vi "PDF Protokoll O2 Leaktest.vi"(8 "error in (no error)":errorcluster caption="Fehler (Eingang, kein Fehler)") -> (0 "error out":errorcluster caption="Fehler (Ausgang)")   [LabVIEW 2020, in "O2 Dichtheitstest.lvlib"]
uses:
  O2 Dichtheitstest.lvlib
  Seiten/System Einstellungen V2/Aktioen FGV System Konstanten.ctl
  Aktion FGV O2 Leak.ctl
  <vilib>/Utility/miscctls.llb/LVPrintingMarginsTypeDef.ctl
  Allgemein/allgemeine Sub-VIs.lvlib
  Seiten/System Einstellungen V2/System Einstellungen V2.lvlib
panel:
  out "Grenzwert Messgasdruck:":string
  out "Messgasdruck:":string
  out "Grenzwert O2:":string
  out "Bestanden":bool caption="Boolesch"
  out "Nullgas Messwert:":string
  out "Datenerfassungszeit:":string
  out "Nullgas Aufschaltzeit:":string
  out "Analysator:":string
  out "Aufschaltpunkt:":string
  out "Endzeit:":string
  out "Startzeit:":string
  out "Ser.Nr.:":string caption="Serien Nummer:"
  out "Messgerät:":string
  # "O2 Leaktest"
  # "s"
  # "s"
  # "kPa"
  # "%"
  # "IAG-Industrie Automatisierungsgeschellschaft m.b.H.    l  Industriestraße 2    l    2722Weikersdorf     )+43262221734 7+43262221734655"
  # "kPa"
  # "%"
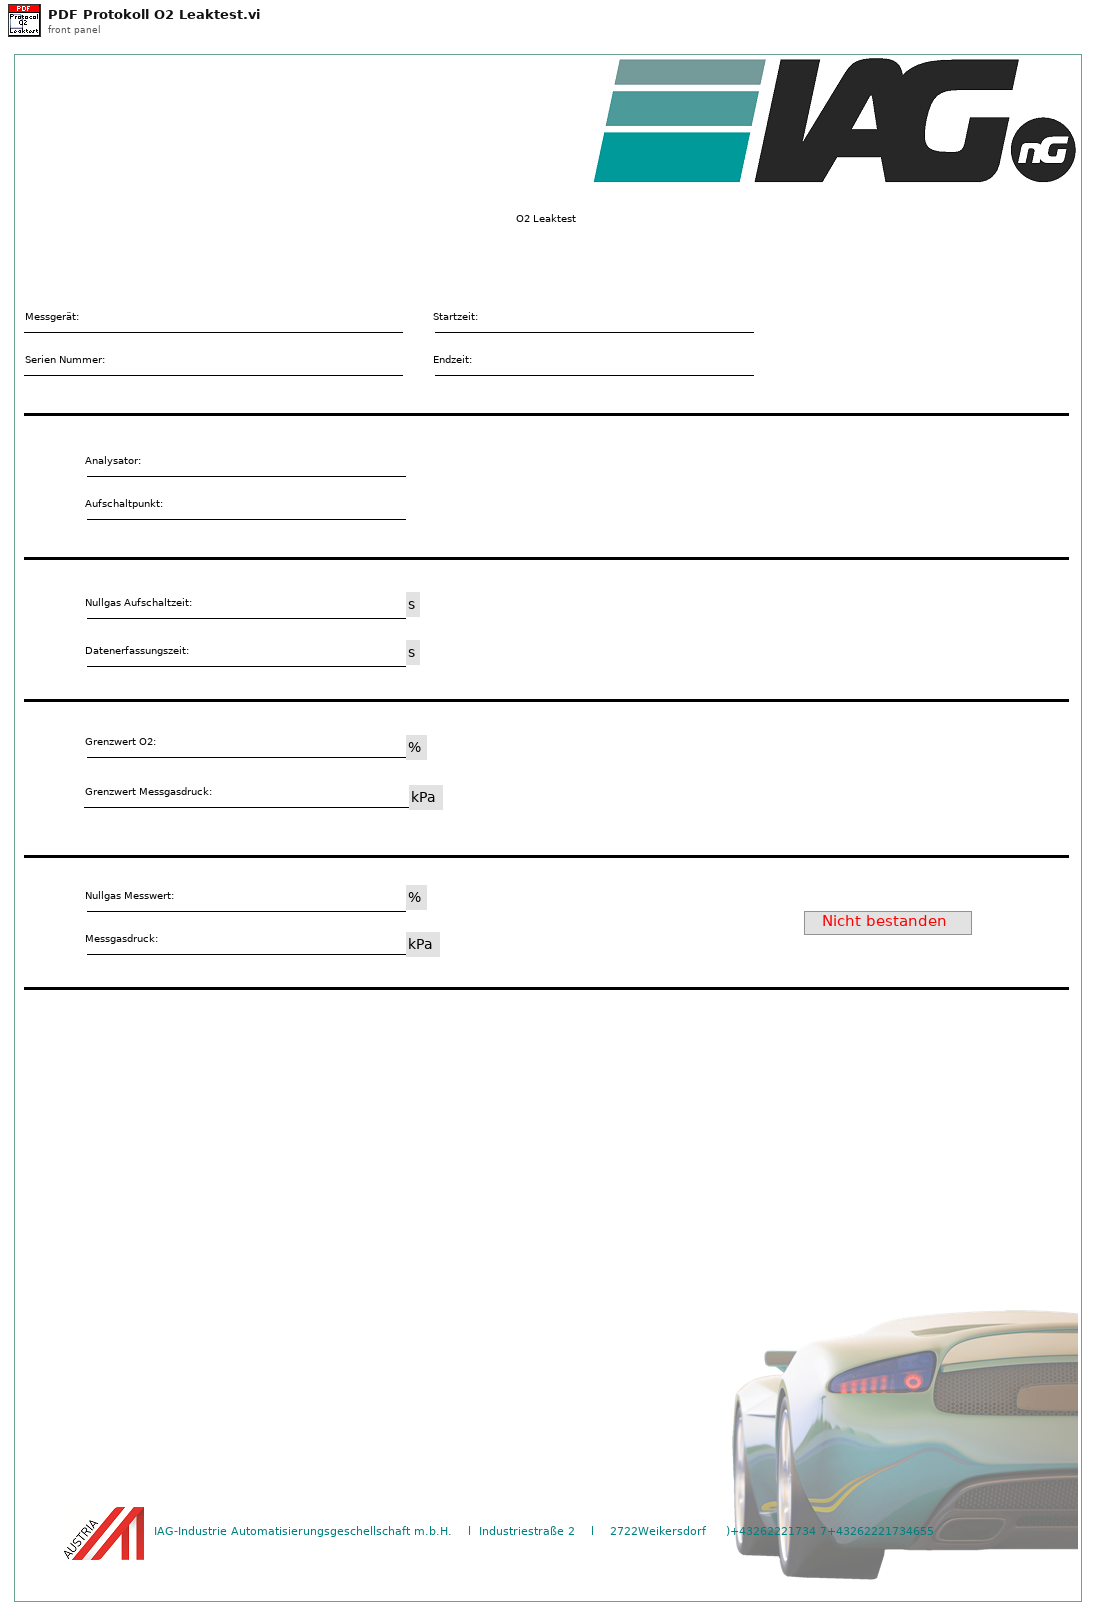
[diagram p1: front panel]
types:
  T1 = typedef "O2 Dichtheitstest.lvlib/Aktion FGV O2 Leak.ctl" = enum16{"lesen", "O2 settings", "Pfad", "Protokoll", "laden", "speichern"}
  T2 = typedef "System Einstellungen V2.lvlib/Aktioen FGV System Konstanten.ctl" = enum16{"lesen", "laden", "speichern", "Sprache"}
  T3 = enum32{"Portrait", "Landscape", "Rotated Portrait", "Rotated Landscape"}
  T4 = typedef "LVPrintingMarginsTypeDef.ctl" = cluster{"Top":sgl, "Left":sgl, "Bottom":sgl, "Right":sgl, "Measurement System":enum8{"Inches", "cm"}}
  T5 = typedef "O2 Dichtheitstest.lvlib/O2 Settings.ctl" = cluster{"Kalibriergas":T6, "Aufschaltpunkt":T6, "Nullgas Aufschaltzeit:":sgl, "Datenerfassungszeit:":sgl, "Grenzwert: O2":sgl, "Grenzwert: Messgasdruck":sgl, "Grenzwert: Messgasdruck 2":sgl}
  T6 = typedef "Auswahlfeld.ctl" = u16
  T7 = typedef "O2 Dichtheitstest.lvlib/Protokoll LeakTest.ctl" = cluster{"O2":sgl, "Messgasdruck":sgl, "Startzeit":timestamp, "Endzeit":timestamp, "Bestanden?":bool}
  T8 = cluster{"Modell":string, "ProjektNummer":string, "Software Version":string, "Seriennummer":string}
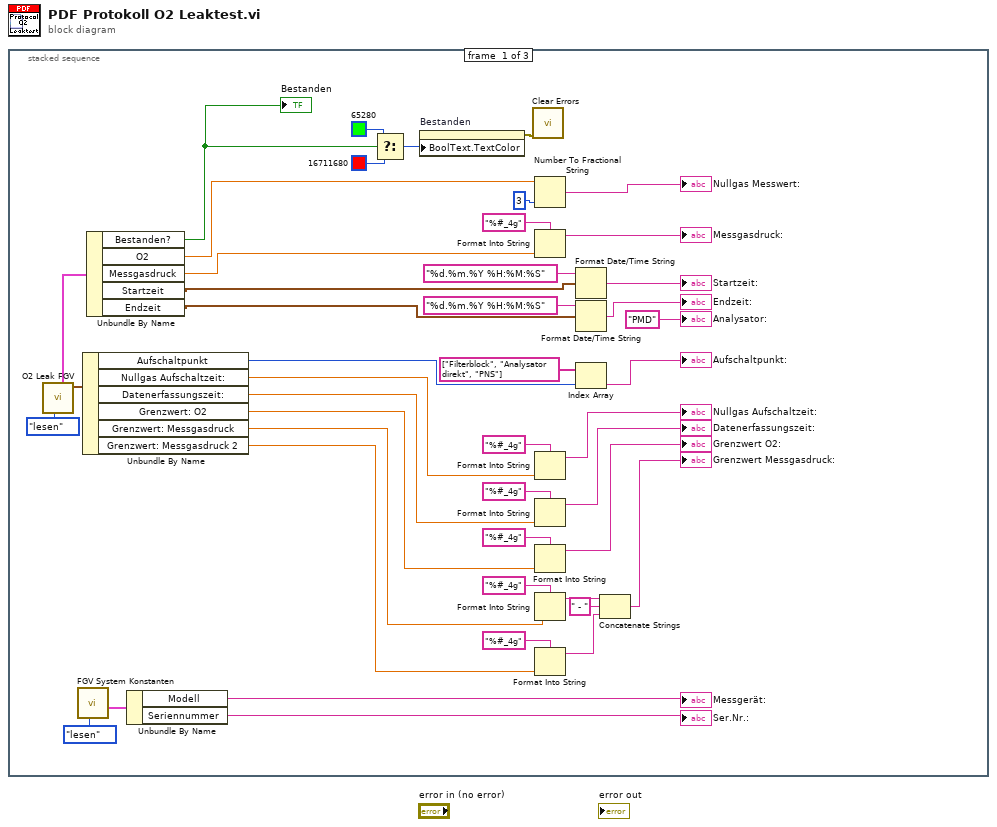
[diagram p0: block diagram]
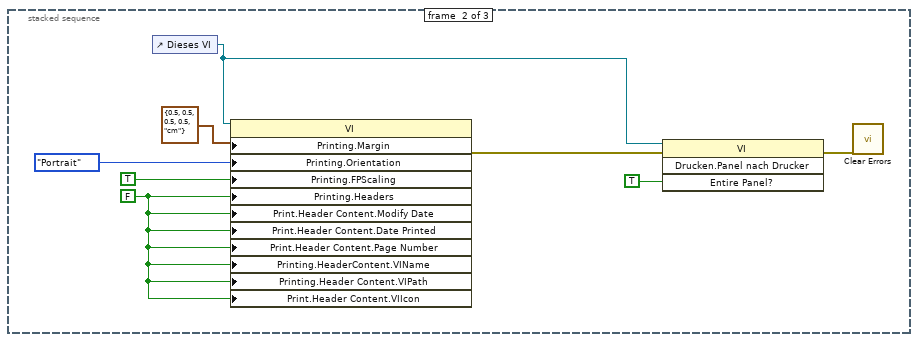
[diagram p2: hidden frame]
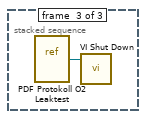
[diagram p3: hidden frame]
diagram:
  n1 = stacked-sequence {
    frame #0 {
      n2 = call "O2 Leak FGV.vi"("Aktion"=Aktion_FGV_O2_Leak."lesen") -> ("O2 Settings"=w17:T5, "Protokoll"=w18:T7)  [unwired: 6 in, 3 out]
      n3 = call "FGV System Konstanten.vi"("Aktionen"=Aktioen_FGV_System_Konstanten."lesen") -> ("Cluster out"=w44:T8)  [unwired: 6 in, 4 out]
      n4 = Unbundle By Name(w17) -> ("Aufschaltpunkt"=w14:T6, "Nullgas Aufschaltzeit:"=w12:sgl, "Datenerfassungszeit:"=w11:sgl, "Grenzwert: O2"=w10:sgl, "Grenzwert: Messgasdruck"=w9:sgl, "Grenzwert: Messgasdruck 2"=w7:sgl)
      n5 = Unbundle By Name(w18) -> ("Bestanden?"=w8:bool, "O2"=w1:sgl, "Messgasdruck"=w13:sgl, "Startzeit"=w16:timestamp, "Endzeit"=w15:timestamp)
      "Bestanden" <- w8
      n6 = Unbundle By Name(w44) -> ("Modell"=→"Messgerät:":string, "Seriennummer"=→"Ser.Nr.:":string)
      n7 = Select(t=u32 65280, s=w8, f=u32 16711680) -> (s? t:f=w21:u32)
      n8 = property on="Bestanden" class="Bool. (strikt)"("BoolText.TextColor"=w21) -> (error out=w20:errorcluster)  [unwired: 2 in, 1 out]
      n9 = call <vilib>:"Clear Errors.vi"("error in (no error)"=w20) -> ()  [unwired: 5 in, 2 out]
      n10 = Number To Fractional String(number=w1, precision (6)=i16 3 ("Breite (-)")) -> (F-format string=→"Nullgas Messwert:":string)  [unwired: 2 in]
      n11 = Format Into String(format string="%#_4g" ("Format-String"), w13) -> (resulting string=→"Messgasdruck:":string)  [unwired: 2 in, 1 out]
      n12 = Format Into String(format string="%#_4g" ("Format-String"), w12) -> (resulting string=→"Nullgas Aufschaltzeit:":string)  [unwired: 2 in, 1 out]
      n13 = Format Into String(format string="%#_4g" ("Format-String"), w11) -> (resulting string=→"Datenerfassungszeit:":string)  [unwired: 2 in, 1 out]
      n14 = Format Into String(format string="%#_4g" ("Format-String"), w10) -> (resulting string=→"Grenzwert O2:":string)  [unwired: 2 in, 1 out]
      n15 = Format Into String(format string="%#_4g" ("Format-String"), w9) -> (resulting string=w27:string)  [unwired: 2 in, 1 out]
      n16 = Format Into String(format string="%#_4g" ("Format-String"), w7) -> (resulting string=w5:string)  [unwired: 2 in, 1 out]
      n17 = Format Date/Time String(time format string (%c)="%d.%m.%Y %H:%M:%S" ("Zeitformatierungs-String (%c)"), seconds (now)=w16) -> (date/time string=→"Startzeit:":string)  [unwired: 1 in]
      n18 = Format Date/Time String(time format string (%c)="%d.%m.%Y %H:%M:%S" ("Zeitformatierungs-String (%c)"), seconds (now)=w15) -> (date/time string=→"Endzeit:":string)  [unwired: 1 in]
      n19 = Index Array(array=string[] ["Filterblock", "Analysator direkt", "PNS"], index=w14) -> (element=→"Aufschaltpunkt:":string)
      n20 = Concatenate Strings(w27, " - " ("String"), w5) -> (→"Grenzwert Messgasdruck:":string)
      "Analysator:" <- "PMD" ("Analysator:")
    }
    frame #1 {
      w48 = FALSE ("Drucken:Kopfzeilen?")
      n21 = control-ref of="Dieses VI"() -> (w51:refnum<vi>)
      n22 = property class="VI"(reference=w51, "Printing.Margin"=T4 {"Top"=0.5, "Left"=0.5, "Bottom"=0.5, "Right"=0.5, "Measurement System"=enum."cm"} ("Drucken:Ränder"), "Printing.Orientation"=T3."Portrait" ("Drucken:Seitenausrichtung"), "Printing.FPScaling"=TRUE ("Drucken:Frontpanel-Skalierung?"), "Printing.Headers"=w48, "Print.Header Content.Modify Date"=w48, "Print.Header Content.Date Printed"=w48, "Print.Header Content.Page Number"=w48, "Printing.HeaderContent.VIName"=w48, "Printing.Header Content.VIPath"=w48, "Print.Header Content.VIIcon"=w48) -> (error out=w53:errorcluster)  [unwired: 1 in, 1 out]
      n23 = invoke class="VI" method="Drucken.Panel nach Drucker"(reference=w51, error in=w53, "Entire Panel?"=TRUE ("Abschnittskopfzeilen?")) -> (error out=w46:errorcluster)  [unwired: 1 in, 3 out]
      n24 = call <vilib>:"Clear Errors.vi"("error in (no error)"=w46) -> ()  [unwired: 5 in, 2 out]
    }
    frame #2 {
      n25 = vi-ref "PDF Protokoll O2 Leaktest.vi"() -> (w54:refnum<vi>)
      n26 = call "VI Shut Down.vi"("VI Referenz"=w54) -> ()  [unwired: 11 in]
    }
  }
